vi "DO Write.vi"(8 "error in":errorcluster, 10 "DO data":bool[][](array[boolean])=[[TRUE, TRUE, FALSE, TRUE], [TRUE, TRUE, TRUE, FALSE], [TRUE, FALSE, FALSE, FALSE], [TRUE, FALSE, FALSE, FALSE], [TRUE, FALSE, FALSE, FALSE]], 11 "task/channels in":refnum<k21>[](array[refnum])) -> (0 "Array":errorcluster[](array[cluster]))   [LabVIEW 2022 SP3]
uses:
  <vilib>/DAQmx/write.llb/DAQmx Write (Digital 1D Bool NChan 1Samp 1Line).vi
  <vilib>/DAQmx/miscellaneous.llb/DAQmx Fill In Error Info.vi
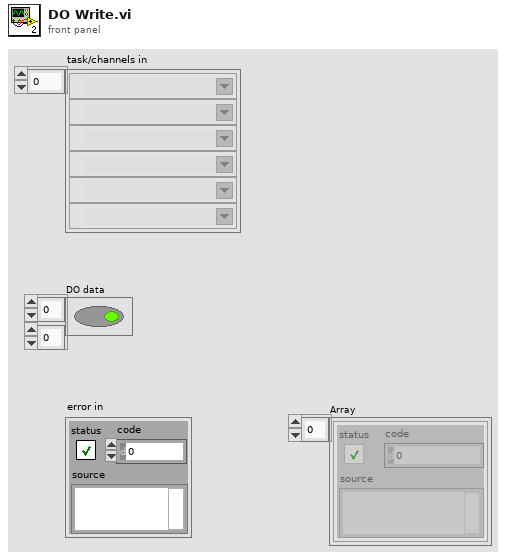
[diagram p1: front panel]
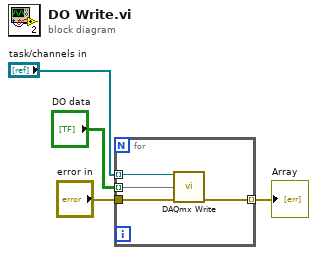
[diagram p0: block diagram]
diagram:
  n1 = for {
    tunnel: "task/channels in" -> [w8] mode=indexing
    tunnel: "DO data" -> [w7] mode=indexing
    tunnel: [w6] -> w3 mode=indexing
    tunnel: "error in" -> [w5]
    n2 = call-poly <vilib>:"DAQmx Write.vi"("task/channels in"=w8, "data"=w7, "error in"=w5) -> ("error out"=w6:errorcluster)  [unwired: 10 in, 2 out]
  }
  "Array" <- w3
